vi "Servo demo.vi"() -> ()   [LabVIEW 2018]
uses:
  <vilib>/myRIO/Common/Instrument Driver Framework/myRIO v1.0/PWM/vis/myRIO v1.1 Open PWM.vi
  <vilib>/myRIO/Common/Instrument Driver Framework/myRIO v1.0/UART/vis/myRIO v1.0 Close UART.vi
  <vilib>/myRIO/Common/Instrument Driver Framework/Utilities/vis/Validate Channels.vi
  <vilib>/myRIO/Common/Instrument Driver Framework/myRIO v1.0/PWM/vis/myRIO v1.0 Reserve PWM.vi
  <vilib>/myRIO/Common/Instrument Driver Framework/myRIO v1.0/PWM/vis/myRIO v1.0 Build MUX Configuration PWM.vi
  <vilib>/myRIO/Common/Instrument Driver Framework/myRIO v1.0/Resource Manager/vis/myRIO v1.0 Reserve Channel List.vi
  <vilib>/myRIO/Common/Instrument Driver Framework/myRIO v1.0/Resource Manager/vis/myRIO v1.0 Create Configuration List.vi
  <vilib>/myRIO/Common/Instrument Driver Framework/myRIO v1.0/Resource Manager/vis/myRIO v1.0 Reserve Channel.vi
  <vilib>/myRIO/Common/Instrument Driver Framework/myRIO v1.0/Resource Manager/vis/myRIO v1.0 Unreserve Channel.vi
  <vilib>/myRIO/Common/Instrument Driver Framework/myRIO v1.0/Resource Manager/vis/myRIO v1.0 Build Mutex Name.vi
  <vilib>/Utility/VariantDataType/GetNumericInfo.vi
  <vilib>/Utility/error.llb/Error Cluster From Error Code.vi
  <vilib>/myRIO/Common/Instrument Driver Framework/myRIO v1.0/myRIO v1.1 Open.vi
  <vilib>/myRIO/Common/Instrument Driver Framework/Utilities/vis/IO Manager.vi
  <vilib>/myRIO/Common/Instrument Driver Framework/Utilities/vis/Configuration Manager.vi
  <vilib>/myRIO/Common/Instrument Driver Framework/myRIO v1.0/Resource Manager/vis/myRIO v1.0 Configure IO.vi
  <vilib>/myRIO/Common/Instrument Driver Framework/myRIO v1.0/myRIO v1.0 Close.vi
  <vilib>/myRIO/Common/Instrument Driver Framework/myRIO v1.0/PWM/vis/myRIO v1.0 Write PWM.vi
  <vilib>/myRIO/Common/Instrument Driver Framework/Utilities/vis/FPGA Ref Manager.vi
  <vilib>/myRIO/Common/Instrument Driver Framework/myRIO v1.0/myRIO v1.0 Reset FPGA.vi
  <vilib>/myRIO/Common/Instrument Driver Framework/myRIO v1.0/IRQ/vis/myRIO v1.0 IRQ Info FGV.vi
  <vilib>/myRIO/Common/Instrument Driver Framework/myRIO v1.0/IRQ/vis/myRIO v1.0 Timer IRQ Info FGV.vi
  <vilib>/myRIO/Common/Instrument Driver Framework/myRIO v1.0/IRQ/vis/myRIO v1.0 ISR Agent.vi
  <vilib>/myRIO/Instrument Drivers/Utilities/Utilities.lvlib
  <vilib>/myRIO/Instrument Drivers/Onboard IO/PWM/PWM.lvlib
panel:
  out "offset [%FS]":dbl
  in  "null offset":bool
  out "duty cycle [%]":dbl
  out "pulse width [ms]":dbl=1.5
  in  "freq [Hz]":dbl=50.0
  in  "PWM channel":tag="B/PWM0"
  in  "position [%FS]":dbl(slide) scale=-200.0..200.0
  in  "[ESC]":bool
  # "Servo demo"
  # "Brun -gnd\nRød - 5V\nOrange - PWM"
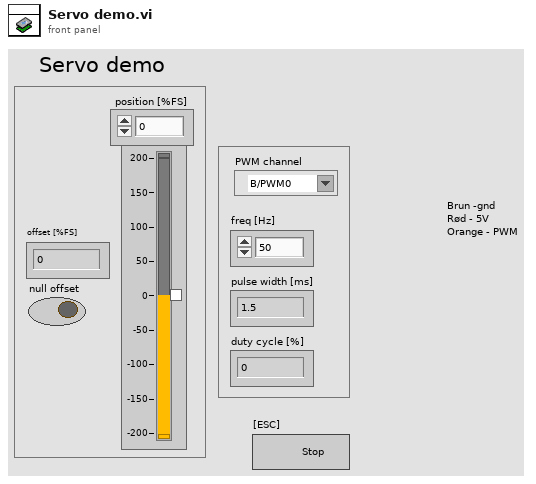
[diagram p1: front panel]
types:
  T1 = typedef "PWM.lvlib/PWM Reference.ctl" = cluster{"myRIO Reference":T2, "PWM Channels Enum":T6, "PWM Configuration":T7}
  T2 = typedef "myRIO Generic Hardware Reference.ctl" = cluster{"myRIO Model":T3, "myRIO Hardware Reference":T4}
  T3 = typedef "Hardware Version Enum.ctl" = enum16{"Unknown", "myRIO-1900", "myRIO-1950", "roboRIO", "NI ELVIS RIO CM", "ELVIS III"}
  T4 = typedef "myRIO v1.0 Reference.ctl" = cluster{"Generic FPGA Reference":T5, "Allow multiple opens":bool}
  T5 = typedef "Generic FPGA Reference.ctl" = refnum<k20>
  T6 = typedef "PWM Channels Enum.ctl" = enum16{"Not Connected", "C/PWM0", "C/PWM1", "A/PWM0", "A/PWM1", "A/PWM2", "A/PWM3", "A/PWM4", "A/PWM5", "A/PWM6", "A/PWM7", "A/PWM8", "A/PWM9", "A/PWM10", "A/PWM11", "A/PWM12", "A/PWM13", "A/PWM14", "A/PWM15", "A/PWM16", "A/PWM17", "A/PWM18", "A/PWM19", "B/PWM0", "B/PWM1", "B/PWM2", "B/PWM3", "B/PWM4", "B/PWM5", "B/PWM6", "B/PWM7", "B/PWM8", "B/PWM9", "B/PWM10", "B/PWM11", "B/PWM12", "B/PWM13", "B/PWM14", "B/PWM15", "B/PWM16", "B/PWM17", "B/PWM18", "B/PWM19", "PWM/PWM0", "PWM/PWM1", "PWM/PWM2", "PWM/PWM3", "PWM/PWM4", "PWM/PWM5", "PWM/PWM6", "PWM/PWM7", "PWM/PWM8", "PWM/PWM9"}
  T7 = typedef "PWM.lvlib/PWM Configuration.ctl" = cluster{"Frequency":dbl, "Duty Cycle":dbl}
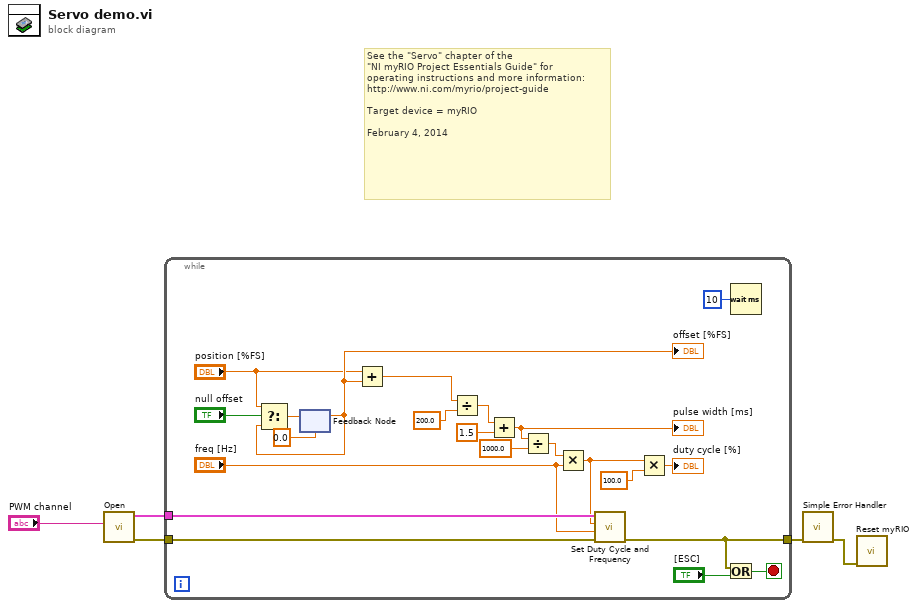
[diagram p0: block diagram]
diagram:
  # "See the \"Servo\" chapter of the\n\"NI myRIO Project Essentials Guide\" for\noperating instructions and more information: \nhttp://www.ni.com/myrio/project-guide\n\nTarget device = myRIO\n\nFebruary 4, 2014"
  n1 = call <vilib>:"Open.vi"("Channel Name"="PWM channel") -> ("error out"=w2:errorcluster, "PWM Ref Out"=w3:T1)  [unwired: 9 in]
  n2 = while {
    tunnel: w3 -> [w19]
    tunnel: w2 -> [w18]
    tunnel: [w16] -> w1
    stop <- w27 stop-if-true
    n3 = feedback #1(0.0 ("position [%FS]")) -> (w12:dbl)
    "offset [%FS]" <- w12
    n4 = Select(t="position [%FS]", s="null offset", f=w12) -> (s? t:f=w14:dbl)
    n5 = feedback-in #1(w14) -> ()
    n6 = Add(x="position [%FS]", y=w12) -> (x+y=w13:dbl)
    n7 = Divide(x=w13, y=200.0) -> (x/y=w23:dbl)
    n8 = Add(x=w23, y=1.5) -> (x+y=w21:dbl)
    "pulse width [ms]" <- w21
    n9 = Divide(x=w21, y=1000.0) -> (x/y=w10:dbl)
    n10 = Multiply(x=w10, y="freq [Hz]") -> (x*y=w7:dbl)
    n11 = call <vilib>:"Set Duty Cycle and Frequency.vi"("error in (no error)"=w18, "Frequency [Hz]"="freq [Hz]", "Duty Cycle"=w7, "PWM Ref In"=w19) -> ("error out"=w16:errorcluster)  [unwired: 5 in, 1 out]
    n12 = Multiply(x=w7, y=100.0) -> (x*y=→"duty cycle [%]":dbl)
    n13 = Or(x=w16, y="[ESC]") -> (x .or. y?=w27:bool)
    n14 = Wait (ms)(milliseconds to wait=u32 10) -> ()  [unwired: 1 out]
  }
  n15 = call <vilib>:"Simple Error Handler.vi"("error in (no error)"=w1) -> ("error out"=w5:errorcluster)  [unwired: 4 in, 4 out]
  n16 = call <vilib>:"Reset myRIO.vi"("error in (no error)"=w5) -> ()  [unwired: 10 in, 1 out]
